vi "Coloured_Dot_Plotting.vi"(1 "JobVectorDirectory":path, 2 "Data":string[][](array[string]), 3 "Template Filename":path, 4 "Channel Names":string[](array[string])) -> ()   [LabVIEW 2021]
uses:
  Controls/Group_Binning.ctl
  Data_File_Type.ctl
panel:
  in  "Moving Z":u16(ring) items=["Date Sortable", "Rig", "Run Command File", "Run Start Time", "Run Description", "Row Number", "Row Type", "Row Start (sec)", "Row Comment", "Timestamp", "Time In Row(s)", "Config", "Config Num", "Errata", "Omit", "WD", "WD.Pt", "WD.Pt.Cfg", "Point ID", "Point Row", "Legend0", "Downrange Distance (ft)", "Point Height Num", "Point Column", "Legend1", "- MeasuredVariables -----------", "-- VelocityStats --", "U_{dem} Nominal (m/s)", "U_{ref} (m/s)", "Uref ADAM (m/s)", "\\overline{U_{raw}} /U_{ref}", "U_{ref} ADAM /U_{ref}", "\\overline{U} (m/s)", "U corr (m/s)", "\\overline{V} (m/s)", "\\overline{W} (m/s)", "\\overline{|UV|} (m/s)", "\\overline{|UW|} (m/s)", "\\overline{|UVW|} (m/s)", "\\overline{\\theta} (deg)", "\\sigma^2(U) (m/s)^2", "\\sigma^2(V) (m/s)^2", "\\sigma^2(W) (m/s)^2", "\\sigma^2(|UV|) (m/s)^2", "\\sigma^2(|UW|) (m/s)^2", "\\sigma^2(|UVW|) (m/s)^2", "\\sigma^2(\\theta) (deg^2)", "u'v' (m^2/s^2)", "v'w' (m^2/s^2)", "u'w' (m^2/s^2)", "-- VelocityStatsEnd --", "-- QAstats --", "Omni meanPSU (V)", "Omni varPSU (V^2)", "Omni Cal Slope", "Omni Cal Intercept", "Temp (C)", "No Of Measurement Blocks", "No of Analogue Samples", "Flow Measurement Time", "Decimation", "AFRaw nGood perDecBlock", "AFGoodV nGood perDecBlock", "AFGoodVP nGood perDecBlock", "AFRaw nCone<58 deg", "AFRaw nCone<90 deg", "AFRaw Cone<58 deg", "AFRaw Cone<90 deg", "Run Messages", "-- QAstatsEnd --", "- MeasuredVariablesEnd -----------", "Max (ConeAngle) (deg)", "Valid AFReduction Fraction", "Valid Velocity Fraction", "Valid 5hpPressure Fraction", "- LocationsStart -------------", "Scale", "Probe Angle (deg)", "Row X 0", "X (mm)", "Y (mm)", "Z (mm)", "U_{ref} Z (mm)", "Metadata Motor X", "Metadata Motor Y", "Metadata Motor Z", "- LocationsEnd -------------", "- BLsetupBlock ------------", "BLS Trip[1] Ach(mm)", "BLS Trip[2] Ach(mm)", "BLS Spires[1] Ach(mm)", "BLS Spires[1]TipJoint Ach(mm)", "BLS Spires[1] Tips(mm)", "BLS Spires[2] Ach(mm)", "BLS Main[1] Ach(mm)", "BLS Main[2] Ach(mm)", "BLS Main[3] Ach(mm)", "BLS Boost[1] Ach(mm)", "BLS Boost[2] Ach(mm)", "BLS Boost[3] Ach(mm)", "Main Avg (mm)", "Boost Avg (mm)", "Spires[1] Total (mm)", "Ramp Request 0", "Ramp Request 1", "Ramp Request 2", "Ramp Request 3", "Ramp Request 4", "Ramp Request 5", "Ramp Request 6", "Ramp Request 7", "Ramp Request 8", "Ramp Request 9", "Ramp Request 10", "Ramp Request 11", "Ramp Request 12", "FORMATTED OUTPUT BELOW-THIS-------------", "Configuration", "Wind Direction (deg)", "BL Setup", "PointID", "Uref (m/s)", "Mean U /U_{ref}", "Mean V /U_{ref}", "Mean W /U_{ref}", "Mean |UV| /U_{ref}", "Mean |UW| /U_ref", "Mean |UVW| /U_ref", "Yaw (UV) (deg)", "TI (U) (/U)", "TI (U) (/|UV|)", "TI (V) (/|UV|)", "TI (W) (/|UW|)", "TI (|UV|) (/|UV|)", "TI (|UW|) (/|UW|)", "TI (|UVW|) (/|UVW|)", "TI Joint (%)", "Velocity Validation (percent)", "Raw Data Filename", "FORMATTED OUTPUT ABOVE-THIS---------------", "Current File", "Current Filepath", "Template File Used", "Seconds since 1st Jan", "Point Row Column", "Row Y", "X (in)", "Y (in)", "Z (in)", "STL name"]
  in  "Moving Y":u16(ring) items=["Date Sortable", "Rig", "Run Command File", "Run Start Time", "Run Description", "Row Number", "Row Type", "Row Start (sec)", "Row Comment", "Timestamp", "Time In Row(s)", "Config", "Config Num", "Errata", "Omit", "WD", "WD.Pt", "WD.Pt.Cfg", "Point ID", "Point Row", "Legend0", "Downrange Distance (ft)", "Point Height Num", "Point Column", "Legend1", "- MeasuredVariables -----------", "-- VelocityStats --", "U_{dem} Nominal (m/s)", "U_{ref} (m/s)", "Uref ADAM (m/s)", "\\overline{U_{raw}} /U_{ref}", "U_{ref} ADAM /U_{ref}", "\\overline{U} (m/s)", "U corr (m/s)", "\\overline{V} (m/s)", "\\overline{W} (m/s)", "\\overline{|UV|} (m/s)", "\\overline{|UW|} (m/s)", "\\overline{|UVW|} (m/s)", "\\overline{\\theta} (deg)", "\\sigma^2(U) (m/s)^2", "\\sigma^2(V) (m/s)^2", "\\sigma^2(W) (m/s)^2", "\\sigma^2(|UV|) (m/s)^2", "\\sigma^2(|UW|) (m/s)^2", "\\sigma^2(|UVW|) (m/s)^2", "\\sigma^2(\\theta) (deg^2)", "u'v' (m^2/s^2)", "v'w' (m^2/s^2)", "u'w' (m^2/s^2)", "-- VelocityStatsEnd --", "-- QAstats --", "Omni meanPSU (V)", "Omni varPSU (V^2)", "Omni Cal Slope", "Omni Cal Intercept", "Temp (C)", "No Of Measurement Blocks", "No of Analogue Samples", "Flow Measurement Time", "Decimation", "AFRaw nGood perDecBlock", "AFGoodV nGood perDecBlock", "AFGoodVP nGood perDecBlock", "AFRaw nCone<58 deg", "AFRaw nCone<90 deg", "AFRaw Cone<58 deg", "AFRaw Cone<90 deg", "Run Messages", "-- QAstatsEnd --", "- MeasuredVariablesEnd -----------", "Max (ConeAngle) (deg)", "Valid AFReduction Fraction", "Valid Velocity Fraction", "Valid 5hpPressure Fraction", "- LocationsStart -------------", "Scale", "Probe Angle (deg)", "Row X 0", "X (mm)", "Y (mm)", "Z (mm)", "U_{ref} Z (mm)", "Metadata Motor X", "Metadata Motor Y", "Metadata Motor Z", "- LocationsEnd -------------", "- BLsetupBlock ------------", "BLS Trip[1] Ach(mm)", "BLS Trip[2] Ach(mm)", "BLS Spires[1] Ach(mm)", "BLS Spires[1]TipJoint Ach(mm)", "BLS Spires[1] Tips(mm)", "BLS Spires[2] Ach(mm)", "BLS Main[1] Ach(mm)", "BLS Main[2] Ach(mm)", "BLS Main[3] Ach(mm)", "BLS Boost[1] Ach(mm)", "BLS Boost[2] Ach(mm)", "BLS Boost[3] Ach(mm)", "Main Avg (mm)", "Boost Avg (mm)", "Spires[1] Total (mm)", "Ramp Request 0", "Ramp Request 1", "Ramp Request 2", "Ramp Request 3", "Ramp Request 4", "Ramp Request 5", "Ramp Request 6", "Ramp Request 7", "Ramp Request 8", "Ramp Request 9", "Ramp Request 10", "Ramp Request 11", "Ramp Request 12", "FORMATTED OUTPUT BELOW-THIS-------------", "Configuration", "Wind Direction (deg)", "BL Setup", "PointID", "Uref (m/s)", "Mean U /U_{ref}", "Mean V /U_{ref}", "Mean W /U_{ref}", "Mean |UV| /U_{ref}", "Mean |UW| /U_ref", "Mean |UVW| /U_ref", "Yaw (UV) (deg)", "TI (U) (/U)", "TI (U) (/|UV|)", "TI (V) (/|UV|)", "TI (W) (/|UW|)", "TI (|UV|) (/|UV|)", "TI (|UW|) (/|UW|)", "TI (|UVW|) (/|UVW|)", "TI Joint (%)", "Velocity Validation (percent)", "Raw Data Filename", "FORMATTED OUTPUT ABOVE-THIS---------------", "Current File", "Current Filepath", "Template File Used", "Seconds since 1st Jan", "Point Row Column", "Row Y", "X (in)", "Y (in)", "Z (in)", "STL name"]
  in  "Moving X":u16(ring) items=["Date Sortable", "Rig", "Run Command File", "Run Start Time", "Run Description", "Row Number", "Row Type", "Row Start (sec)", "Row Comment", "Timestamp", "Time In Row(s)", "Config", "Config Num", "Errata", "Omit", "WD", "WD.Pt", "WD.Pt.Cfg", "Point ID", "Point Row", "Legend0", "Downrange Distance (ft)", "Point Height Num", "Point Column", "Legend1", "- MeasuredVariables -----------", "-- VelocityStats --", "U_{dem} Nominal (m/s)", "U_{ref} (m/s)", "Uref ADAM (m/s)", "\\overline{U_{raw}} /U_{ref}", "U_{ref} ADAM /U_{ref}", "\\overline{U} (m/s)", "U corr (m/s)", "\\overline{V} (m/s)", "\\overline{W} (m/s)", "\\overline{|UV|} (m/s)", "\\overline{|UW|} (m/s)", "\\overline{|UVW|} (m/s)", "\\overline{\\theta} (deg)", "\\sigma^2(U) (m/s)^2", "\\sigma^2(V) (m/s)^2", "\\sigma^2(W) (m/s)^2", "\\sigma^2(|UV|) (m/s)^2", "\\sigma^2(|UW|) (m/s)^2", "\\sigma^2(|UVW|) (m/s)^2", "\\sigma^2(\\theta) (deg^2)", "u'v' (m^2/s^2)", "v'w' (m^2/s^2)", "u'w' (m^2/s^2)", "-- VelocityStatsEnd --", "-- QAstats --", "Omni meanPSU (V)", "Omni varPSU (V^2)", "Omni Cal Slope", "Omni Cal Intercept", "Temp (C)", "No Of Measurement Blocks", "No of Analogue Samples", "Flow Measurement Time", "Decimation", "AFRaw nGood perDecBlock", "AFGoodV nGood perDecBlock", "AFGoodVP nGood perDecBlock", "AFRaw nCone<58 deg", "AFRaw nCone<90 deg", "AFRaw Cone<58 deg", "AFRaw Cone<90 deg", "Run Messages", "-- QAstatsEnd --", "- MeasuredVariablesEnd -----------", "Max (ConeAngle) (deg)", "Valid AFReduction Fraction", "Valid Velocity Fraction", "Valid 5hpPressure Fraction", "- LocationsStart -------------", "Scale", "Probe Angle (deg)", "Row X 0", "X (mm)", "Y (mm)", "Z (mm)", "U_{ref} Z (mm)", "Metadata Motor X", "Metadata Motor Y", "Metadata Motor Z", "- LocationsEnd -------------", "- BLsetupBlock ------------", "BLS Trip[1] Ach(mm)", "BLS Trip[2] Ach(mm)", "BLS Spires[1] Ach(mm)", "BLS Spires[1]TipJoint Ach(mm)", "BLS Spires[1] Tips(mm)", "BLS Spires[2] Ach(mm)", "BLS Main[1] Ach(mm)", "BLS Main[2] Ach(mm)", "BLS Main[3] Ach(mm)", "BLS Boost[1] Ach(mm)", "BLS Boost[2] Ach(mm)", "BLS Boost[3] Ach(mm)", "Main Avg (mm)", "Boost Avg (mm)", "Spires[1] Total (mm)", "Ramp Request 0", "Ramp Request 1", "Ramp Request 2", "Ramp Request 3", "Ramp Request 4", "Ramp Request 5", "Ramp Request 6", "Ramp Request 7", "Ramp Request 8", "Ramp Request 9", "Ramp Request 10", "Ramp Request 11", "Ramp Request 12", "FORMATTED OUTPUT BELOW-THIS-------------", "Configuration", "Wind Direction (deg)", "BL Setup", "PointID", "Uref (m/s)", "Mean U /U_{ref}", "Mean V /U_{ref}", "Mean W /U_{ref}", "Mean |UV| /U_{ref}", "Mean |UW| /U_ref", "Mean |UVW| /U_ref", "Yaw (UV) (deg)", "TI (U) (/U)", "TI (U) (/|UV|)", "TI (V) (/|UV|)", "TI (W) (/|UW|)", "TI (|UV|) (/|UV|)", "TI (|UW|) (/|UW|)", "TI (|UVW|) (/|UVW|)", "TI Joint (%)", "Velocity Validation (percent)", "Raw Data Filename", "FORMATTED OUTPUT ABOVE-THIS---------------", "Current File", "Current Filepath", "Template File Used", "Seconds since 1st Jan", "Point Row Column", "Row Y", "X (in)", "Y (in)", "Z (in)", "STL name"]
  in  "Scalar":u16(ring) items=["Date Sortable", "Rig", "Run Command File", "Run Start Time", "Run Description", "Row Number", "Row Type", "Row Start (sec)", "Row Comment", "Timestamp", "Time In Row(s)", "Config", "Config Num", "Errata", "Omit", "WD", "WD.Pt", "WD.Pt.Cfg", "Point ID", "Point Row", "Legend0", "Downrange Distance (ft)", "Point Height Num", "Point Column", "Legend1", "- MeasuredVariables -----------", "-- VelocityStats --", "U_{dem} Nominal (m/s)", "U_{ref} (m/s)", "Uref ADAM (m/s)", "\\overline{U_{raw}} /U_{ref}", "U_{ref} ADAM /U_{ref}", "\\overline{U} (m/s)", "U corr (m/s)", "\\overline{V} (m/s)", "\\overline{W} (m/s)", "\\overline{|UV|} (m/s)", "\\overline{|UW|} (m/s)", "\\overline{|UVW|} (m/s)", "\\overline{\\theta} (deg)", "\\sigma^2(U) (m/s)^2", "\\sigma^2(V) (m/s)^2", "\\sigma^2(W) (m/s)^2", "\\sigma^2(|UV|) (m/s)^2", "\\sigma^2(|UW|) (m/s)^2", "\\sigma^2(|UVW|) (m/s)^2", "\\sigma^2(\\theta) (deg^2)", "u'v' (m^2/s^2)", "v'w' (m^2/s^2)", "u'w' (m^2/s^2)", "-- VelocityStatsEnd --", "-- QAstats --", "Omni meanPSU (V)", "Omni varPSU (V^2)", "Omni Cal Slope", "Omni Cal Intercept", "Temp (C)", "No Of Measurement Blocks", "No of Analogue Samples", "Flow Measurement Time", "Decimation", "AFRaw nGood perDecBlock", "AFGoodV nGood perDecBlock", "AFGoodVP nGood perDecBlock", "AFRaw nCone<58 deg", "AFRaw nCone<90 deg", "AFRaw Cone<58 deg", "AFRaw Cone<90 deg", "Run Messages", "-- QAstatsEnd --", "- MeasuredVariablesEnd -----------", "Max (ConeAngle) (deg)", "Valid AFReduction Fraction", "Valid Velocity Fraction", "Valid 5hpPressure Fraction", "- LocationsStart -------------", "Scale", "Probe Angle (deg)", "Row X 0", "X (mm)", "Y (mm)", "Z (mm)", "U_{ref} Z (mm)", "Metadata Motor X", "Metadata Motor Y", "Metadata Motor Z", "- LocationsEnd -------------", "- BLsetupBlock ------------", "BLS Trip[1] Ach(mm)", "BLS Trip[2] Ach(mm)", "BLS Spires[1] Ach(mm)", "BLS Spires[1]TipJoint Ach(mm)", "BLS Spires[1] Tips(mm)", "BLS Spires[2] Ach(mm)", "BLS Main[1] Ach(mm)", "BLS Main[2] Ach(mm)", "BLS Main[3] Ach(mm)", "BLS Boost[1] Ach(mm)", "BLS Boost[2] Ach(mm)", "BLS Boost[3] Ach(mm)", "Main Avg (mm)", "Boost Avg (mm)", "Spires[1] Total (mm)", "Ramp Request 0", "Ramp Request 1", "Ramp Request 2", "Ramp Request 3", "Ramp Request 4", "Ramp Request 5", "Ramp Request 6", "Ramp Request 7", "Ramp Request 8", "Ramp Request 9", "Ramp Request 10", "Ramp Request 11", "Ramp Request 12", "FORMATTED OUTPUT BELOW-THIS-------------", "Configuration", "Wind Direction (deg)", "BL Setup", "PointID", "Uref (m/s)", "Mean U /U_{ref}", "Mean V /U_{ref}", "Mean W /U_{ref}", "Mean |UV| /U_{ref}", "Mean |UW| /U_ref", "Mean |UVW| /U_ref", "Yaw (UV) (deg)", "TI (U) (/U)", "TI (U) (/|UV|)", "TI (V) (/|UV|)", "TI (W) (/|UW|)", "TI (|UV|) (/|UV|)", "TI (|UW|) (/|UW|)", "TI (|UVW|) (/|UVW|)", "TI Joint (%)", "Velocity Validation (percent)", "Raw Data Filename", "FORMATTED OUTPUT ABOVE-THIS---------------", "Current File", "Current Filepath", "Template File Used", "Seconds since 1st Jan", "Point Row Column", "Row Y", "X (in)", "Y (in)", "Z (in)", "STL name"]
  in  "Fixed Z":u16(ring) items=["Date Sortable", "Rig", "Run Command File", "Run Start Time", "Run Description", "Row Number", "Row Type", "Row Start (sec)", "Row Comment", "Timestamp", "Time In Row(s)", "Config", "Config Num", "Errata", "Omit", "WD", "WD.Pt", "WD.Pt.Cfg", "Point ID", "Point Row", "Legend0", "Downrange Distance (ft)", "Point Height Num", "Point Column", "Legend1", "- MeasuredVariables -----------", "-- VelocityStats --", "U_{dem} Nominal (m/s)", "U_{ref} (m/s)", "Uref ADAM (m/s)", "\\overline{U_{raw}} /U_{ref}", "U_{ref} ADAM /U_{ref}", "\\overline{U} (m/s)", "U corr (m/s)", "\\overline{V} (m/s)", "\\overline{W} (m/s)", "\\overline{|UV|} (m/s)", "\\overline{|UW|} (m/s)", "\\overline{|UVW|} (m/s)", "\\overline{\\theta} (deg)", "\\sigma^2(U) (m/s)^2", "\\sigma^2(V) (m/s)^2", "\\sigma^2(W) (m/s)^2", "\\sigma^2(|UV|) (m/s)^2", "\\sigma^2(|UW|) (m/s)^2", "\\sigma^2(|UVW|) (m/s)^2", "\\sigma^2(\\theta) (deg^2)", "u'v' (m^2/s^2)", "v'w' (m^2/s^2)", "u'w' (m^2/s^2)", "-- VelocityStatsEnd --", "-- QAstats --", "Omni meanPSU (V)", "Omni varPSU (V^2)", "Omni Cal Slope", "Omni Cal Intercept", "Temp (C)", "No Of Measurement Blocks", "No of Analogue Samples", "Flow Measurement Time", "Decimation", "AFRaw nGood perDecBlock", "AFGoodV nGood perDecBlock", "AFGoodVP nGood perDecBlock", "AFRaw nCone<58 deg", "AFRaw nCone<90 deg", "AFRaw Cone<58 deg", "AFRaw Cone<90 deg", "Run Messages", "-- QAstatsEnd --", "- MeasuredVariablesEnd -----------", "Max (ConeAngle) (deg)", "Valid AFReduction Fraction", "Valid Velocity Fraction", "Valid 5hpPressure Fraction", "- LocationsStart -------------", "Scale", "Probe Angle (deg)", "Row X 0", "X (mm)", "Y (mm)", "Z (mm)", "U_{ref} Z (mm)", "Metadata Motor X", "Metadata Motor Y", "Metadata Motor Z", "- LocationsEnd -------------", "- BLsetupBlock ------------", "BLS Trip[1] Ach(mm)", "BLS Trip[2] Ach(mm)", "BLS Spires[1] Ach(mm)", "BLS Spires[1]TipJoint Ach(mm)", "BLS Spires[1] Tips(mm)", "BLS Spires[2] Ach(mm)", "BLS Main[1] Ach(mm)", "BLS Main[2] Ach(mm)", "BLS Main[3] Ach(mm)", "BLS Boost[1] Ach(mm)", "BLS Boost[2] Ach(mm)", "BLS Boost[3] Ach(mm)", "Main Avg (mm)", "Boost Avg (mm)", "Spires[1] Total (mm)", "Ramp Request 0", "Ramp Request 1", "Ramp Request 2", "Ramp Request 3", "Ramp Request 4", "Ramp Request 5", "Ramp Request 6", "Ramp Request 7", "Ramp Request 8", "Ramp Request 9", "Ramp Request 10", "Ramp Request 11", "Ramp Request 12", "FORMATTED OUTPUT BELOW-THIS-------------", "Configuration", "Wind Direction (deg)", "BL Setup", "PointID", "Uref (m/s)", "Mean U /U_{ref}", "Mean V /U_{ref}", "Mean W /U_{ref}", "Mean |UV| /U_{ref}", "Mean |UW| /U_ref", "Mean |UVW| /U_ref", "Yaw (UV) (deg)", "TI (U) (/U)", "TI (U) (/|UV|)", "TI (V) (/|UV|)", "TI (W) (/|UW|)", "TI (|UV|) (/|UV|)", "TI (|UW|) (/|UW|)", "TI (|UVW|) (/|UVW|)", "TI Joint (%)", "Velocity Validation (percent)", "Raw Data Filename", "FORMATTED OUTPUT ABOVE-THIS---------------", "Current File", "Current Filepath", "Template File Used", "Seconds since 1st Jan", "Point Row Column", "Row Y", "X (in)", "Y (in)", "Z (in)", "STL name"]
  in  "Fixed Y":u16(ring) items=["Date Sortable", "Rig", "Run Command File", "Run Start Time", "Run Description", "Row Number", "Row Type", "Row Start (sec)", "Row Comment", "Timestamp", "Time In Row(s)", "Config", "Config Num", "Errata", "Omit", "WD", "WD.Pt", "WD.Pt.Cfg", "Point ID", "Point Row", "Legend0", "Downrange Distance (ft)", "Point Height Num", "Point Column", "Legend1", "- MeasuredVariables -----------", "-- VelocityStats --", "U_{dem} Nominal (m/s)", "U_{ref} (m/s)", "Uref ADAM (m/s)", "\\overline{U_{raw}} /U_{ref}", "U_{ref} ADAM /U_{ref}", "\\overline{U} (m/s)", "U corr (m/s)", "\\overline{V} (m/s)", "\\overline{W} (m/s)", "\\overline{|UV|} (m/s)", "\\overline{|UW|} (m/s)", "\\overline{|UVW|} (m/s)", "\\overline{\\theta} (deg)", "\\sigma^2(U) (m/s)^2", "\\sigma^2(V) (m/s)^2", "\\sigma^2(W) (m/s)^2", "\\sigma^2(|UV|) (m/s)^2", "\\sigma^2(|UW|) (m/s)^2", "\\sigma^2(|UVW|) (m/s)^2", "\\sigma^2(\\theta) (deg^2)", "u'v' (m^2/s^2)", "v'w' (m^2/s^2)", "u'w' (m^2/s^2)", "-- VelocityStatsEnd --", "-- QAstats --", "Omni meanPSU (V)", "Omni varPSU (V^2)", "Omni Cal Slope", "Omni Cal Intercept", "Temp (C)", "No Of Measurement Blocks", "No of Analogue Samples", "Flow Measurement Time", "Decimation", "AFRaw nGood perDecBlock", "AFGoodV nGood perDecBlock", "AFGoodVP nGood perDecBlock", "AFRaw nCone<58 deg", "AFRaw nCone<90 deg", "AFRaw Cone<58 deg", "AFRaw Cone<90 deg", "Run Messages", "-- QAstatsEnd --", "- MeasuredVariablesEnd -----------", "Max (ConeAngle) (deg)", "Valid AFReduction Fraction", "Valid Velocity Fraction", "Valid 5hpPressure Fraction", "- LocationsStart -------------", "Scale", "Probe Angle (deg)", "Row X 0", "X (mm)", "Y (mm)", "Z (mm)", "U_{ref} Z (mm)", "Metadata Motor X", "Metadata Motor Y", "Metadata Motor Z", "- LocationsEnd -------------", "- BLsetupBlock ------------", "BLS Trip[1] Ach(mm)", "BLS Trip[2] Ach(mm)", "BLS Spires[1] Ach(mm)", "BLS Spires[1]TipJoint Ach(mm)", "BLS Spires[1] Tips(mm)", "BLS Spires[2] Ach(mm)", "BLS Main[1] Ach(mm)", "BLS Main[2] Ach(mm)", "BLS Main[3] Ach(mm)", "BLS Boost[1] Ach(mm)", "BLS Boost[2] Ach(mm)", "BLS Boost[3] Ach(mm)", "Main Avg (mm)", "Boost Avg (mm)", "Spires[1] Total (mm)", "Ramp Request 0", "Ramp Request 1", "Ramp Request 2", "Ramp Request 3", "Ramp Request 4", "Ramp Request 5", "Ramp Request 6", "Ramp Request 7", "Ramp Request 8", "Ramp Request 9", "Ramp Request 10", "Ramp Request 11", "Ramp Request 12", "FORMATTED OUTPUT BELOW-THIS-------------", "Configuration", "Wind Direction (deg)", "BL Setup", "PointID", "Uref (m/s)", "Mean U /U_{ref}", "Mean V /U_{ref}", "Mean W /U_{ref}", "Mean |UV| /U_{ref}", "Mean |UW| /U_ref", "Mean |UVW| /U_ref", "Yaw (UV) (deg)", "TI (U) (/U)", "TI (U) (/|UV|)", "TI (V) (/|UV|)", "TI (W) (/|UW|)", "TI (|UV|) (/|UV|)", "TI (|UW|) (/|UW|)", "TI (|UVW|) (/|UVW|)", "TI Joint (%)", "Velocity Validation (percent)", "Raw Data Filename", "FORMATTED OUTPUT ABOVE-THIS---------------", "Current File", "Current Filepath", "Template File Used", "Seconds since 1st Jan", "Point Row Column", "Row Y", "X (in)", "Y (in)", "Z (in)", "STL name"]
  in  "Fixed X":u16(ring) items=["Date Sortable", "Rig", "Run Command File", "Run Start Time", "Run Description", "Row Number", "Row Type", "Row Start (sec)", "Row Comment", "Timestamp", "Time In Row(s)", "Config", "Config Num", "Errata", "Omit", "WD", "WD.Pt", "WD.Pt.Cfg", "Point ID", "Point Row", "Legend0", "Downrange Distance (ft)", "Point Height Num", "Point Column", "Legend1", "- MeasuredVariables -----------", "-- VelocityStats --", "U_{dem} Nominal (m/s)", "U_{ref} (m/s)", "Uref ADAM (m/s)", "\\overline{U_{raw}} /U_{ref}", "U_{ref} ADAM /U_{ref}", "\\overline{U} (m/s)", "U corr (m/s)", "\\overline{V} (m/s)", "\\overline{W} (m/s)", "\\overline{|UV|} (m/s)", "\\overline{|UW|} (m/s)", "\\overline{|UVW|} (m/s)", "\\overline{\\theta} (deg)", "\\sigma^2(U) (m/s)^2", "\\sigma^2(V) (m/s)^2", "\\sigma^2(W) (m/s)^2", "\\sigma^2(|UV|) (m/s)^2", "\\sigma^2(|UW|) (m/s)^2", "\\sigma^2(|UVW|) (m/s)^2", "\\sigma^2(\\theta) (deg^2)", "u'v' (m^2/s^2)", "v'w' (m^2/s^2)", "u'w' (m^2/s^2)", "-- VelocityStatsEnd --", "-- QAstats --", "Omni meanPSU (V)", "Omni varPSU (V^2)", "Omni Cal Slope", "Omni Cal Intercept", "Temp (C)", "No Of Measurement Blocks", "No of Analogue Samples", "Flow Measurement Time", "Decimation", "AFRaw nGood perDecBlock", "AFGoodV nGood perDecBlock", "AFGoodVP nGood perDecBlock", "AFRaw nCone<58 deg", "AFRaw nCone<90 deg", "AFRaw Cone<58 deg", "AFRaw Cone<90 deg", "Run Messages", "-- QAstatsEnd --", "- MeasuredVariablesEnd -----------", "Max (ConeAngle) (deg)", "Valid AFReduction Fraction", "Valid Velocity Fraction", "Valid 5hpPressure Fraction", "- LocationsStart -------------", "Scale", "Probe Angle (deg)", "Row X 0", "X (mm)", "Y (mm)", "Z (mm)", "U_{ref} Z (mm)", "Metadata Motor X", "Metadata Motor Y", "Metadata Motor Z", "- LocationsEnd -------------", "- BLsetupBlock ------------", "BLS Trip[1] Ach(mm)", "BLS Trip[2] Ach(mm)", "BLS Spires[1] Ach(mm)", "BLS Spires[1]TipJoint Ach(mm)", "BLS Spires[1] Tips(mm)", "BLS Spires[2] Ach(mm)", "BLS Main[1] Ach(mm)", "BLS Main[2] Ach(mm)", "BLS Main[3] Ach(mm)", "BLS Boost[1] Ach(mm)", "BLS Boost[2] Ach(mm)", "BLS Boost[3] Ach(mm)", "Main Avg (mm)", "Boost Avg (mm)", "Spires[1] Total (mm)", "Ramp Request 0", "Ramp Request 1", "Ramp Request 2", "Ramp Request 3", "Ramp Request 4", "Ramp Request 5", "Ramp Request 6", "Ramp Request 7", "Ramp Request 8", "Ramp Request 9", "Ramp Request 10", "Ramp Request 11", "Ramp Request 12", "FORMATTED OUTPUT BELOW-THIS-------------", "Configuration", "Wind Direction (deg)", "BL Setup", "PointID", "Uref (m/s)", "Mean U /U_{ref}", "Mean V /U_{ref}", "Mean W /U_{ref}", "Mean |UV| /U_{ref}", "Mean |UW| /U_ref", "Mean |UVW| /U_ref", "Yaw (UV) (deg)", "TI (U) (/U)", "TI (U) (/|UV|)", "TI (V) (/|UV|)", "TI (W) (/|UW|)", "TI (|UV|) (/|UV|)", "TI (|UW|) (/|UW|)", "TI (|UVW|) (/|UVW|)", "TI Joint (%)", "Velocity Validation (percent)", "Raw Data Filename", "FORMATTED OUTPUT ABOVE-THIS---------------", "Current File", "Current Filepath", "Template File Used", "Seconds since 1st Jan", "Point Row Column", "Row Y", "X (in)", "Y (in)", "Z (in)", "STL name"]
  in  "OK Button":bool
  in  "Row Selector":i32(listbox)=1
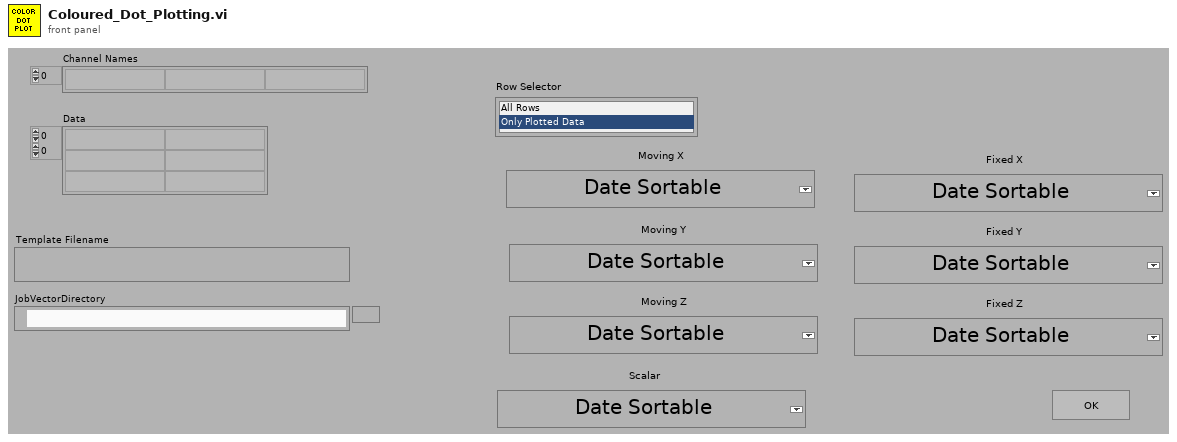
[diagram p1: front panel]
types:
  T1 = typedef "Data_File_Type.ctl" = enum16{"Read All File Types", "Results Files Only", "Raw Data Files Only", "Calibration Files Only", "Gas Desk Files Only", "Old Results Files Only", "Tabulated Data Files Only"}
  T2 = enum16{"Show only data summary", "Show data summary", "No data summary"}
  T3 = typedef "Group_Binning.ctl" = cluster{"Index":i32, "Tolerance":dbl, "Precision":string}
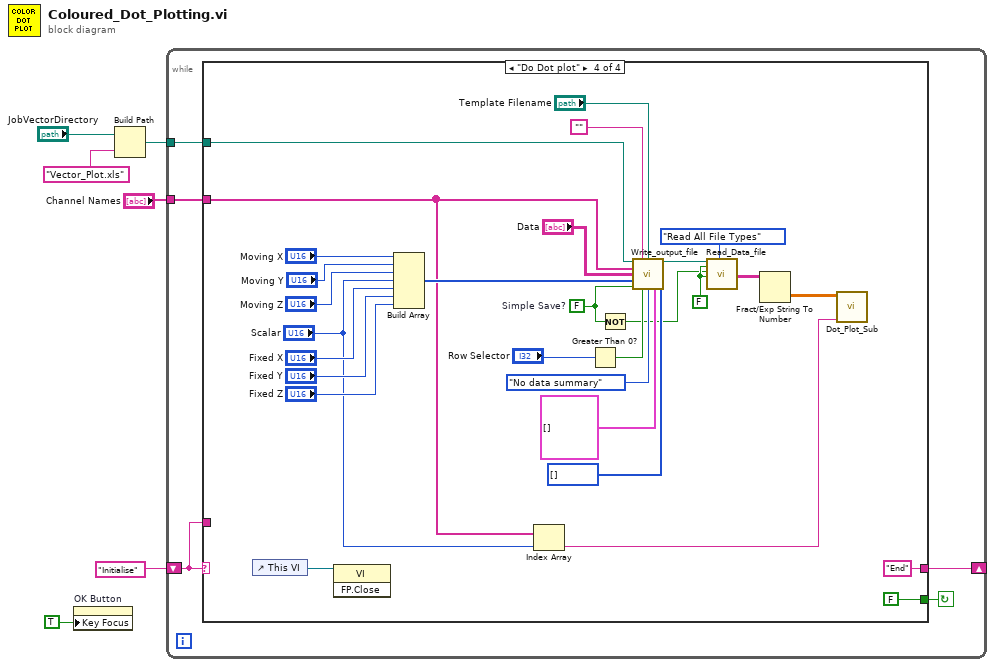
[diagram p0: block diagram]
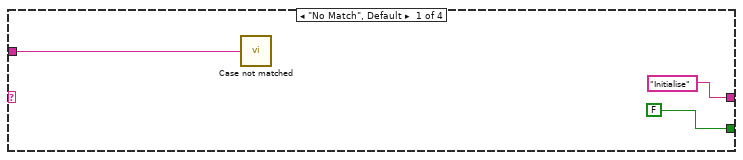
[diagram p2: hidden frame]
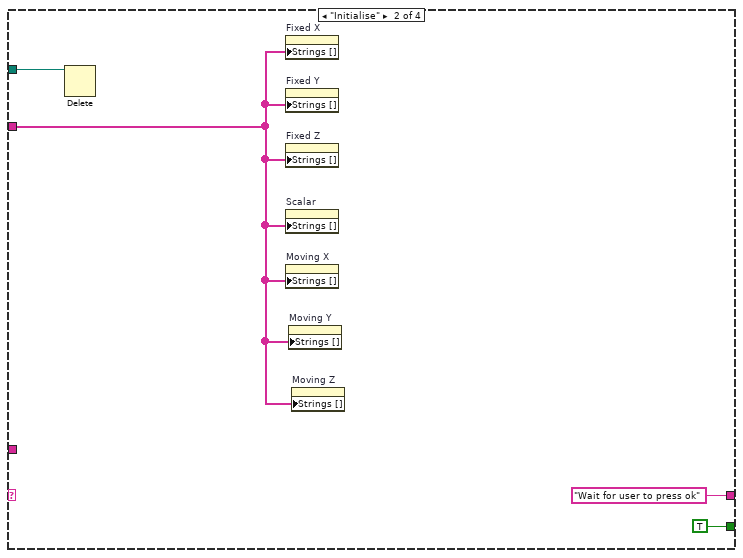
[diagram p3: hidden frame]
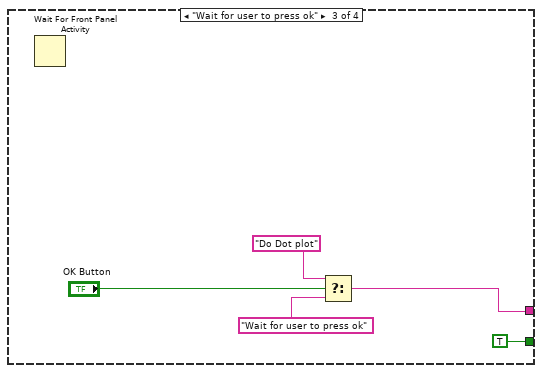
[diagram p4: hidden frame]
diagram:
  n1 = property on="OK Button" class="Bool"("Key Focus"=TRUE) -> ()  [unwired: 2 in, 2 out]
  n2 = Build Path(base path="JobVectorDirectory", name or relative path="Vector_Plot.xls") -> (appended path=w1:path)
  n3 = while {
    shift-left: "Initialise" -> [w9]
    shift-right: [w10] -> _
    tunnel: "Channel Names" -> [w8]
    tunnel: w1 -> [w7]
    stop <- w11 continue-if-true
    n4 = case shown="\"Do Dot plot\"" w9 {
      tunnel: [FALSE TRUE TRUE FALSE] -> w11
      tunnel: ["Initialise" "Wait for user to press ok" w22 "End" ("t")] -> w10
      tunnel: w9 -> [w12 _ _ _]
      tunnel: w8 -> [_ w15 _ w30]
      tunnel: w7 -> [_ w16 _ w40]
      frame "No Match", Default {
        n5 = call "Case not matched.vi"("Case Name not Matched"=w12) -> ()
      }
      frame "Initialise" {
        n6 = Delete(path (use dialog)=w16) -> ()  [unwired: 1 in, 6 out]
        n7 = property on="Fixed X" class="Ring (strict)"("Strings []"=w15) -> ()  [unwired: 2 in, 2 out]
        n8 = property on="Fixed Y" class="Ring (strict)"("Strings []"=w15) -> ()  [unwired: 2 in, 2 out]
        n9 = property on="Fixed Z" class="Ring (strict)"("Strings []"=w15) -> ()  [unwired: 2 in, 2 out]
        n10 = property on="Scalar" class="Ring (strict)"("Strings []"=w15) -> ()  [unwired: 2 in, 2 out]
        n11 = property on="Moving X" class="Ring (strict)"("Strings []"=w15) -> ()  [unwired: 2 in, 2 out]
        n12 = property on="Moving Y" class="Ring (strict)"("Strings []"=w15) -> ()  [unwired: 2 in, 2 out]
        n13 = property on="Moving Z" class="Ring (strict)"("Strings []"=w15) -> ()  [unwired: 2 in, 2 out]
      }
      frame "Wait for user to press ok" {
        n14 = Wait For Front Panel Activity() -> ()  [unwired: 3 in, 1 out]
        n15 = Select(t="Do Dot plot", s="OK Button", f="Wait for user to press ok") -> (s? t:f=w22:string)
      }
      frame "Do Dot plot" {
        w43 = FALSE ("Read Channel Names only")
        w27 = FALSE  # Simple Save?
        n16 = control-ref of="This VI"() -> (w24:refnum<vi>)
        n17 = invoke class="VI" method="FP.Close"(reference=w24) -> ()  [unwired: 2 in, 3 out]
        n18 = Build Array("Moving X", "Moving Y", "Moving Z", "Scalar", "Fixed X", "Fixed Y", "Fixed Z") -> (w31:u16[])
        n19 = Index Array(array=w30, index="Scalar") -> (element=w28:string)
        n20 = Greater Than 0?(x="Row Selector") -> (x > 0?=w46:bool)
        n21 = Not(x=w27) -> (.not. x?=w26:bool)
        n22 = call "Write_output_file.vi"("Output filename"=w40, "Header"="", "Template Filename"="Template Filename", "Channel Names"=w30, "Data"="Data", "Desired Columns"=w31, "Simple Save?"=w27, "Save Plotted rows only?"=w46, "Summarise mode"=T2."No data summary", "Grouping info"=T3[] [], "Channels to Tabulate in header"=i32[] []) -> ("Output filename Out"=w38:path)  [unwired: 1 in, 3 out]
        n23 = call "Read_Data_file.vi"("Results file"=w38, "Read Channel Names only"=w43, "Delete First Rows?"=w26, "Add Extra Channels?"=w43, "Desired File Types"=Data_File_Type."Read All File Types") -> ("Channel Values Out"=w41:string[][])  [unwired: 2 in, 12 out]
        n24 = Fract/Exp String To Number(string=w41) -> (number=w25:dbl[][])  [unwired: 4 out]
        n25 = call "Dot_Plot_Sub.vi"("Scaler plotted"=w28, "Data"=w25) -> ()  [unwired: 10 in]
      }
    }
  }
